vi "Command_Ball_Out.vi"(3 "Timeout":dbl=3.0, 5 "Startup":bool) -> (0 "Speed":dbl, 1 "Completed":bool=TRUE, 2 "Reinit":bool)   [LabVIEW 2018]
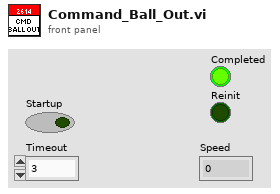
[diagram p1: front panel]
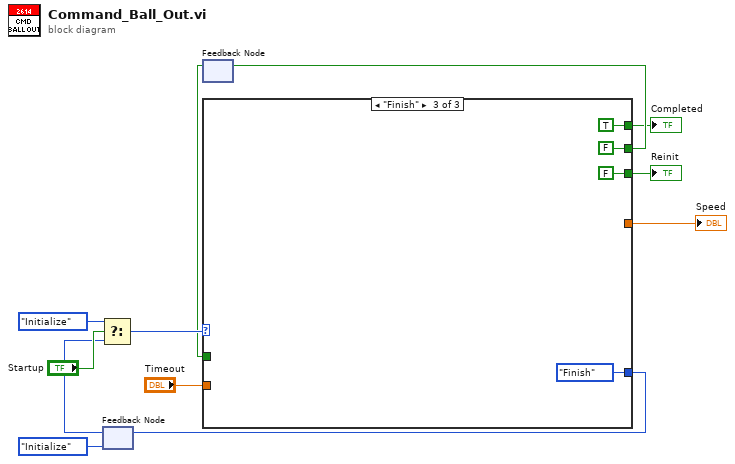
[diagram p0: block diagram]
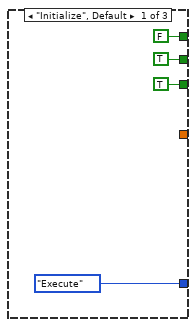
[diagram p2: hidden frame]
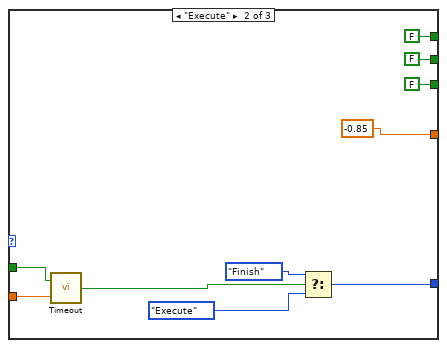
[diagram p3: hidden frame]
diagram:
  n1 = feedback #1(enum16{"Initialize", "Execute", "Finish"}."Initialize" ("f")) -> (w8:enum16{"Initialize", "Execute", "Finish"})
  n2 = Select(t=enum16{"Initialize", "Execute", "Finish"}."Initialize", s="Startup", f=w8) -> (s? t:f=w12:enum16{"Initialize", "Execute", "Finish"})
  n3 = feedback #2() -> (w6:bool)  [unwired: 1 in]
  n4 = case shown="\"Finish\"" w12 {
    tunnel: [enum16{"Initialize", "Execute", "Finish"}."Execute" w23 enum16{"Initialize", "Execute", "Finish"}."Finish" ("f")] -> w9
    tunnel: w6 -> [_ w21 _]
    tunnel: [TRUE FALSE FALSE] -> w7
    tunnel: [FALSE FALSE TRUE] -> w5
    tunnel: [TRUE FALSE FALSE] -> w4
    tunnel: "Timeout" -> [_ w19 _]
    tunnel: [_ -0.85 _] -> w1
    frame "Initialize", Default {
    }
    frame "Execute" {
      n5 = call "Timeout.vi"("Timeout"=w19, "Initialize"=w21) -> ("Timed Out?"=w18:bool)
      n6 = Select(t=enum16{"Initialize", "Execute", "Finish"}."Finish", s=w18, f=enum16{"Initialize", "Execute", "Finish"}."Execute") -> (s? t:f=w23:enum16{"Initialize", "Execute", "Finish"})
    }
    frame "Finish" {
    }
  }
  "Completed" <- w5
  "Reinit" <- w4
  "Speed" <- w1
  n7 = feedback-in #1(w9) -> ()
  n8 = feedback-in #2(w7) -> ()
